vi "aquireUSB650.vi"(6 "Integration Times In":i32[](array[numeric]), 7 "Reference Time":timestamp, 8 "Length of Shot (s)":dbl, 9 "Delay Between Integrations (s)":dbl, 10 "Maximum Number of Integrations":i32, 11 "Wrapper In":u32) -> (1 "Integration Times Out":i32[](array[numeric]), 2 "Time":dbl[](array[numeric]), 3 "Spectrum Values":dbl[][](array[numeric]))   [LabVIEW 2011]
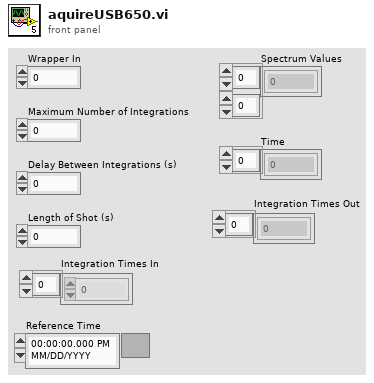
[diagram p1: front panel]
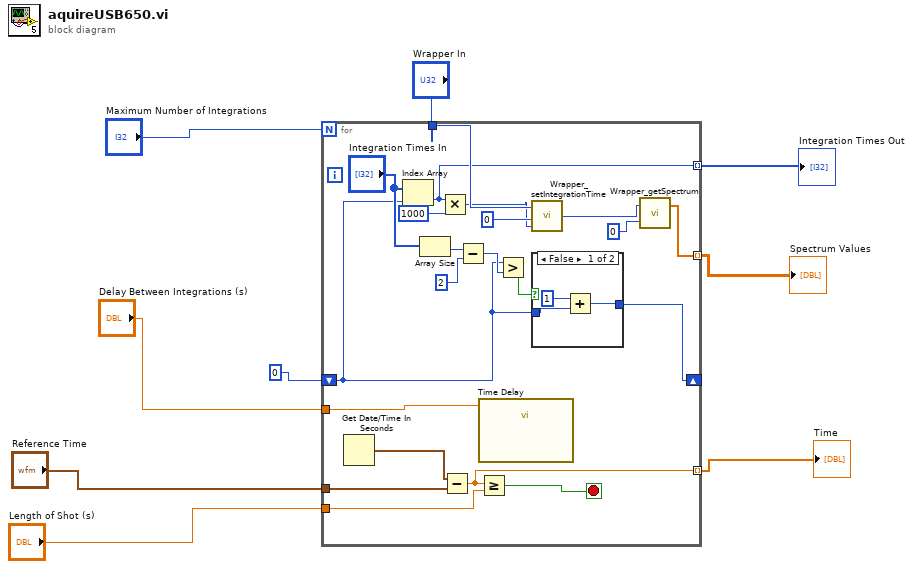
[diagram p0: block diagram]
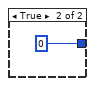
[diagram p2: hidden frame]
diagram:
  n1 = for {
    N: "Maximum Number of Integrations" -> [_]
    tunnel: "Reference Time" -> [w13]
    tunnel: "Length of Shot (s)" -> [w30]
    tunnel: "Wrapper In" -> [w24]
    tunnel: "Delay Between Integrations (s)" -> [w27]
    tunnel: [w25] -> w8 mode=indexing
    tunnel: [w26] -> w9 mode=indexing
    shift-right: [w16] -> _
    shift-left: 0 -> [w15]
    tunnel: [w10] -> w1 mode=indexing
    stop <- w29 stop-if-true
    n2 = Get Date/Time In Seconds() -> (seconds since 1Jan1904=w14:timestamp)
    n3 = Index Array(array="Integration Times In", index=w15) -> (element=w10:i32)
    n4 = Array Size(array="Integration Times In") -> (size(s)=w20:i32)
    n5 = Multiply(x=w10, y=1000) -> (x*y=w11:i32)
    n6 = Subtract(x=w14, y=w13) -> (x-y=w26:dbl)
    n7 = Subtract(x=w20, y=2) -> (x-y=w18:i32)
    n8 = call "Time Delay"("Delay Time (s)"=w27) -> ()  [unwired: 10 in, 1 out]
    n9 = Greater Or Equal?(x=w26, y=w30) -> (x >= y?=w29:bool)
    n10 = Greater?(x=w15, y=w18) -> (0:w17:bool)
    n11 = call "Wrapper_setIntegrationTime.vi"("Integration Time"=w11, "Index"=0, "Wrapper In"=w24) -> ("Wrapper Out"=w23:u32)
    n12 = case shown="False" w17 {
      tunnel: [w32 0] -> w16
      tunnel: w15 -> [w33 _]
      frame False {
        n13 = Add(x=1, y=w33) -> (x+y=w32:i32)
      }
      frame True {
      }
    }
    n14 = call "Wrapper_getSpectrum.vi"("Index"=0, "Wrapper"=w23) -> ("Spectrum Values"=w25:dbl[])  [unwired: 1 out]
  }
  "Time" <- w9
  "Spectrum Values" <- w8
  "Integration Times Out" <- w1
